vi "IMU Get Euler Angle Wrapper.vi"   [LabVIEW 2026, in "MrcLib.lvlib"]
uses:
  MrcLib.lvlib
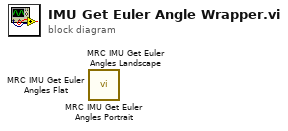
[diagram p0: block diagram]
diagram:
  n1 = call <vilib>:"MRC IMU Get Euler Angles Portrait.vi"() -> ()  [unwired: 9 in, 3 out]
  n2 = call <vilib>:"MRC IMU Get Euler Angles Landscape.vi"() -> ()  [unwired: 9 in, 3 out]
  n3 = call "MRC IMU Get Euler Angles Flat.vi"() -> ()  [unwired: 10 in, 2 out]
